vi "HtmlPrepareHugo.vi"(8 "error in":errorcluster, 10 "ViDescr":string, 11 "Html Path":path) -> (0 "error out":errorcluster)   [LabVIEW 2020]
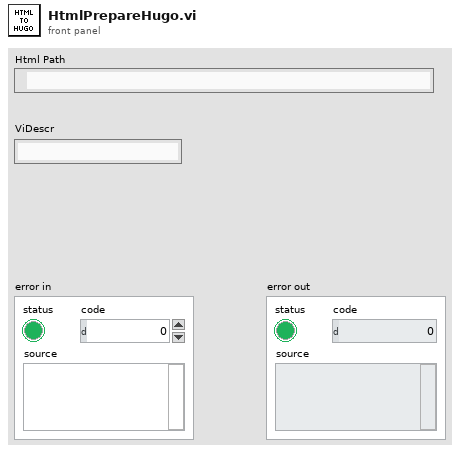
[diagram p1: front panel]
types:
  T1 = enum16{"open", "replace", "create", "open or create", "replace or create", "replace or create with confirmation"}
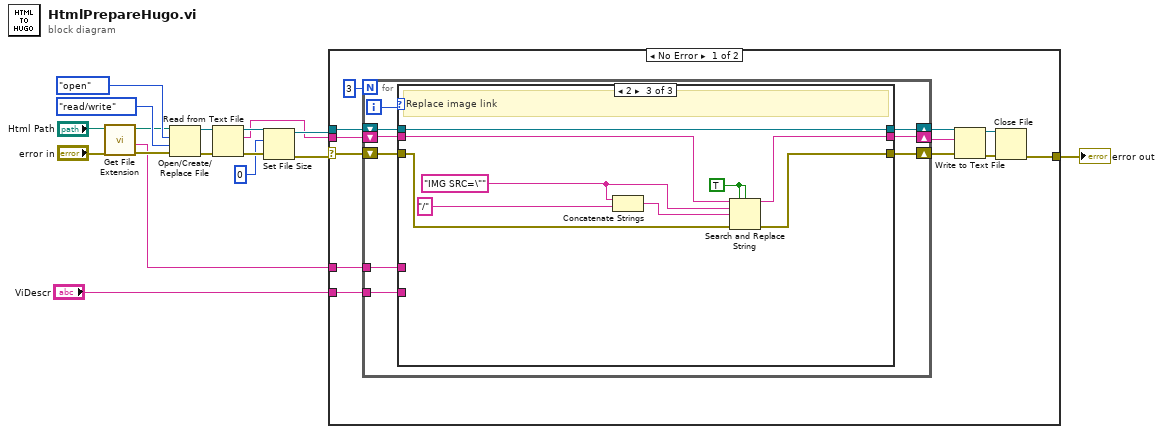
[diagram p0: block diagram]
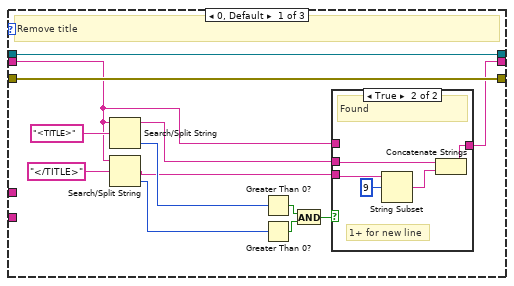
[diagram p2: hidden frame]
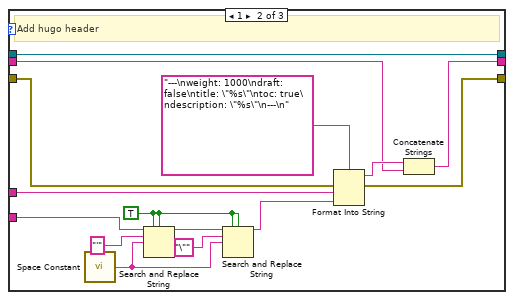
[diagram p4: hidden frame]
diagram:
  n1 = call <vilib>:"Get File Extension.vi"("error in (no error)"="error in", "file"="Html Path") -> ("error out"=w2:errorcluster, "filename without extension"=w1:string, "dup file"=w3:path)  [unwired: 5 in, 2 out]
  n2 = Open/Create/Replace File(file path (use dialog)=w3, error in=w2, operation (0:open)=T1."open", access (0:read/write)=enum16{"read/write", "read-only", "write-only"}."read/write") -> (refnum out=w15:refnum<file>, error out=w16:errorcluster)  [unwired: 2 in, 1 out]
  n3 = Read from Text File(file (use dialog)=w15, error in=w16) -> (refnum out=w11:refnum<file>, text=w7:string, error out=w12:errorcluster)  [unwired: 2 in, 1 out]
  n4 = Set File Size(4:w12, 6:i64 0 ("size (in bytes)"), 7:w11) -> (0:w9:errorcluster, 3:w10:refnum<file>)
  n5 = case shown="No Error" w9 {
    selector: w9 -> [w26 w82]
    tunnel: w7 -> [w29 _]
    tunnel: w10 -> [w27 _]
    tunnel: [w21 w82] -> w17
    tunnel: "ViDescr" -> [w19 _]
    tunnel: w1 -> [w18 _]
    frame No Error {
      n6 = for {
        N: 3 -> [_]
        shift-right: [w32] -> w24
        shift-left: w26 -> [w33]
        shift-right: [w36] -> w20
        shift-left: w27 -> [w37]
        shift-right: [w34] -> w25
        shift-left: w29 -> [w35]
        tunnel: w19 -> [w31]
        tunnel: w18 -> [w30]
        i -> [w38]
        # "remove title"
        n7 = case shown="2" w38 {
          tunnel: w37 -> [w51 w72 w81]
          tunnel: [w51 w72 w81] -> w36
          tunnel: w35 -> [w40 w68 w78]
          tunnel: [w39 w71 w77] -> w34
          tunnel: w33 -> [w48 w65 w80]
          tunnel: [w48 w64 w79] -> w32
          tunnel: w31 -> [_ w62 _]
          tunnel: w30 -> [_ w67 _]
          frame 0, Default {
            # "Remove title"
            n8 = Search/Split String(string=w40, search string/char (-)="<TITLE>") -> (substring before match=w42:string, offset of match=w44:i32)  [unwired: 1 in, 1 out]
            n9 = Search/Split String(string=w40, search string/char (-)="</TITLE>") -> (match + rest of string=w41:string, offset of match=w45:i32)  [unwired: 1 in, 1 out]
            n10 = Greater Than 0?(x=w44) -> (x > 0?=w50:bool)
            n11 = Greater Than 0?(x=w45) -> (x > 0?=w49:bool)
            n12 = And(x=w50, y=w49) -> (x .and. y?=w43:bool)
            n13 = case shown="True" w43 {
              tunnel: w42 -> [_ w55]
              tunnel: w41 -> [_ w57]
              tunnel: w40 -> [w52 _]
              tunnel: [w52 w53] -> w39
              frame False {
                # "not found"
              }
              frame True {
                # "1+ for new line"
                # "Found"
                n14 = String Subset(string=w57, offset (0)=9) -> (substring=w54:string)  [unwired: 1 in]
                n15 = Concatenate Strings(w55, w54) -> (w53:string)
              }
            }
          }
          frame 1 {
            w59 = TRUE
            # "Add hugo header"
            n16 = call <vilib>:"Space Constant.vi"() -> ("String"=w60:string)
            n17 = Search and Replace String(replace all?=w59, case sensitive?=w59, input string=w62, search string="'", replace string=w60) -> (result string=w63:string)  [unwired: 3 in, 3 out]
            n18 = Search and Replace String(replace all?=w59, case sensitive?=w59, input string=w63, search string="\"", replace string=w60) -> (result string=w58:string)  [unwired: 3 in, 3 out]
            n19 = Format Into String(format string="---\nweight: 1000\ndraft: false\ntitle: \"%s\"\ntoc: true\ndescription: \"%s\"\n---\n", error in=w65, w67, w58) -> (resulting string=w69:string, error out=w64:errorcluster)  [unwired: 1 in]
            n20 = Concatenate Strings(w69, w68) -> (w71:string)
          }
          frame 2 {
            w76 = TRUE
            w73 = "IMG SRC=\""
            # "Replace image link"
            n21 = Concatenate Strings(w73, "/") -> (w74:string)
            n22 = Search and Replace String(replace all?=w76, case sensitive?=w76, input string=w78, search string=w73, replace string=w74, error in=w80) -> (result string=w77:string, error out=w79:errorcluster)  [unwired: 2 in, 2 out]
          }
        }
      }
      n23 = Write to Text File(file (use dialog)=w20, text=w25, error in=w24) -> (refnum out=w22:refnum<file>, error out=w23:errorcluster)  [unwired: 1 in, 1 out]
      n24 = Close File(refnum=w22, error in=w23) -> (error out=w21:errorcluster)  [unwired: 1 out]
    }
    frame Error {
    }
  }
  "error out" <- w17
